vi "Call DQMH Scripting Tools.vi"(8 "error in":errorcluster, 9 "DQMH Tools":T2, 10 "Current Selection In":T1, 11 "Project in":refnum<class "Project.lvclass">) -> (0 "error out":errorcluster)   [LabVIEW 2020, in "Panther Dashboard.lvlib"]
uses:
  Panther Dashboard.lvlib
  Class/Project/Project.lvclass
  C:/GitClones/PantherDashboard/src/LabVIEW/Panther Dashboard/Class/LabVIEWItem/LabVIEWItem.lvclass
  DQMH Tools Menu--enum.ctl
  Class/Library/Library.lvclass
  Class/VI/VI.lvclass
  Class/Project/Project.lvclass/Project.ctl
  Class/LabVIEWItem/LabVIEWItem.lvclass/LabVIEWItem.ctl
  Class/LabVIEWItem/Read Item Type.vi
  Class/LabVIEWItem/Read Item Name.vi
  Class/Project/Read Main App Inst Ref.vi
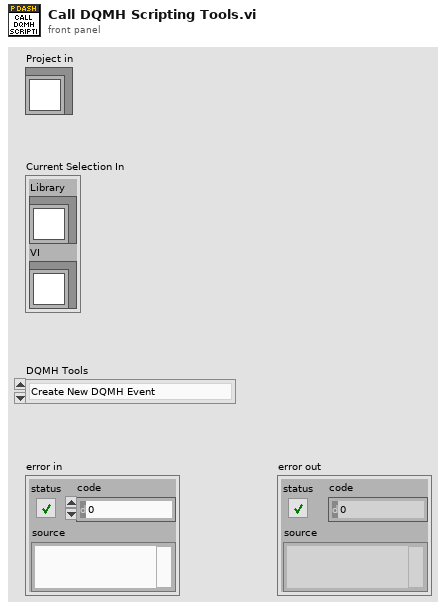
[diagram p1: front panel]
types:
  T1 = cluster{"Library":refnum<class "Library.lvclass">, "VI":refnum<class "VI.lvclass">}
  T2 = typedef "Panther Dashboard.lvlib/DQMH Tools Menu--enum.ctl" = enum16{"Create New DQMH Event", "Remove DQMH Event", "Convert DQMH Event", "Rename DQMH Event", "Add New DQMH Module", "Create RT Tester", "Rename DQMH Module", "Validate DQMH Module", "Create DQMH Module Template", "New DQMH  Unit Test", "Add Helper Loop to DQMH Module", "Duplicate Event", "Duplicate Module"}
  T3 = enum32{"Invalid", "Standard", "Closed", "Hidden", "Minimized", "Maximized"}
  T4 = typedef "Panther Dashboard.lvlib/LabVIEWItem.lvclass/Item Type--enum.ctl" = enum16{"Requests", "Broadcasts", "Request and Wait for Reply", "Round Trip", "» Public API VIs", "» Constant VIs", "» Error VIs", "Module", "Project", "No Drag Selection"}
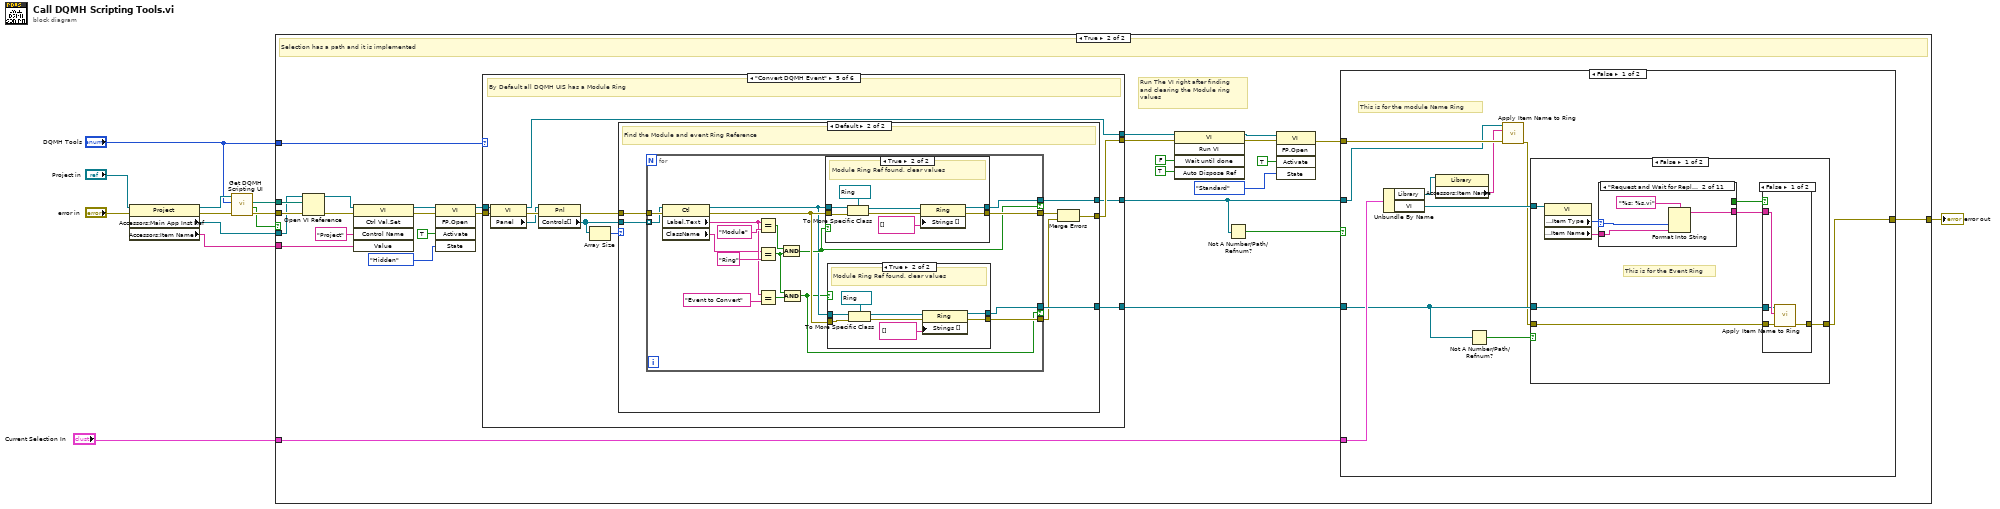
[diagram p0: block diagram]
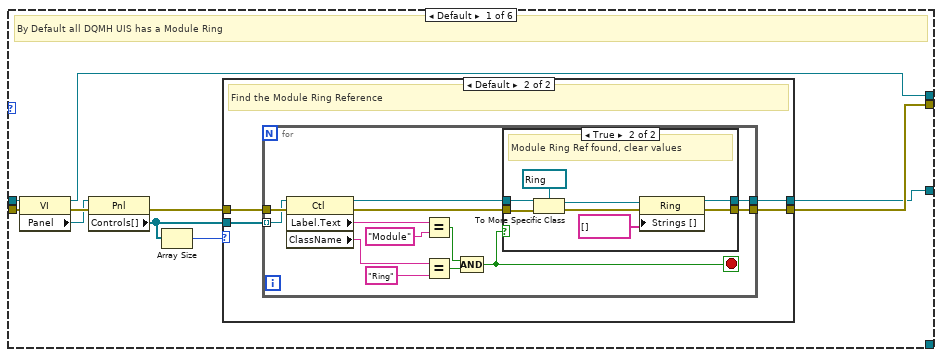
[diagram p3: hidden frame]
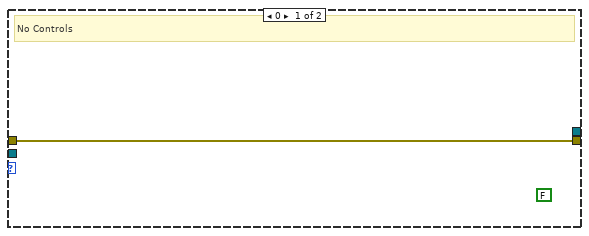
[diagram p4: hidden frame]
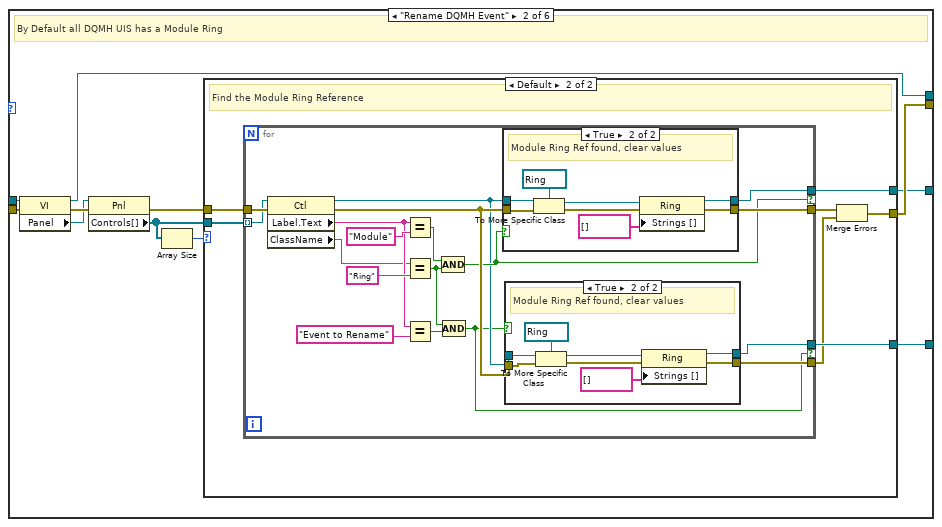
[diagram p6: hidden frame]
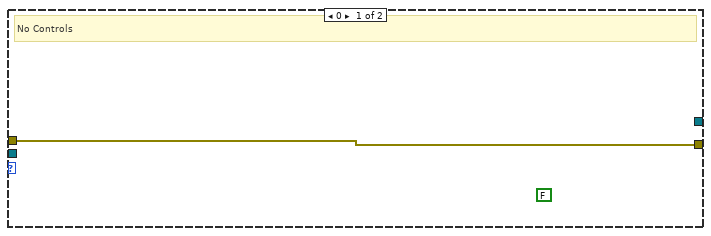
[diagram p7: hidden frame]
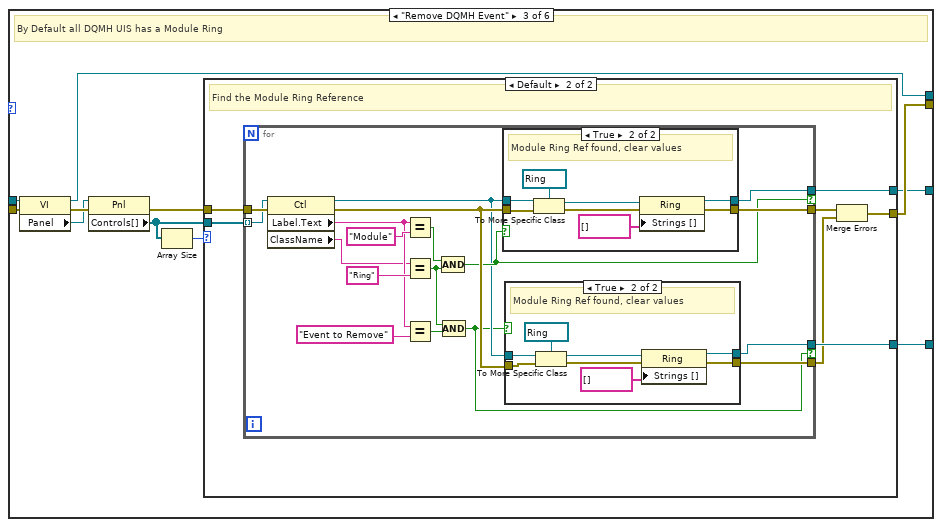
[diagram p10: hidden frame]
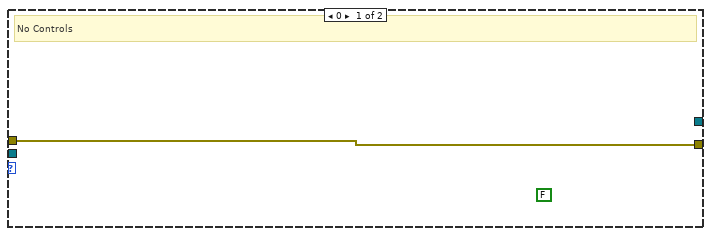
[diagram p11: hidden frame]
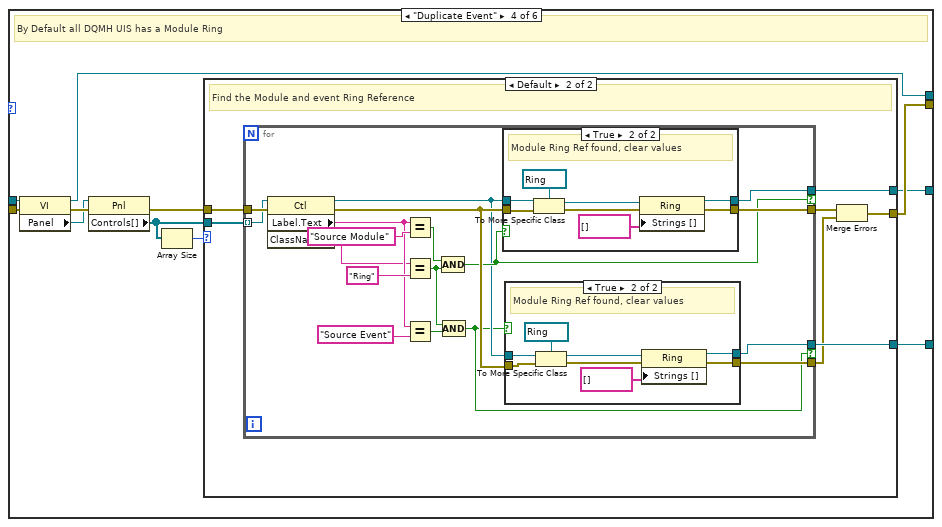
[diagram p14: hidden frame]
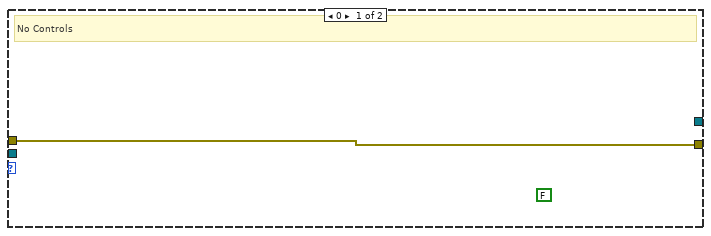
[diagram p15: hidden frame]
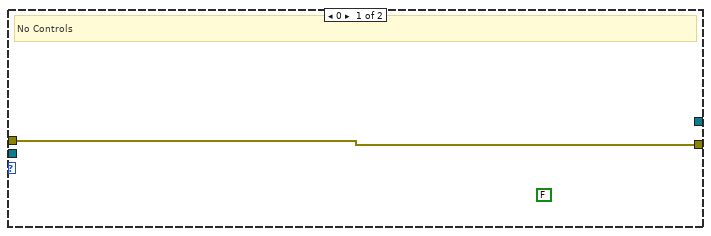
[diagram p18: hidden frame]
diagram:
  n1 = property class="Project"(reference="Project in", error in="error in") -> (reference out=w5:refnum<class "Project.lvclass">, error out=w9:errorcluster, "Accessors:Main App Inst Ref"=w4:refnum<vi>, "Accessors:Item Name"=w3:string)
  n2 = call "Get DQMH Scripting UI.vi"("error in"=w9, "DQMH Tools"="DQMH Tools", "Project in"=w5) -> ("error out"=w12:errorcluster, "Implemented?"=w7:bool, "DQMH UI Path"=w8:path)  [unwired: 6 in]
  n3 = case shown="True" w7 {
    tunnel: w8 -> [_ w32]
    tunnel: w3 -> [_ w27]
    tunnel: [w13 w34] -> w10
    tunnel: w12 -> [w13 w35]
    tunnel: w4 -> [_ w19]
    tunnel: "DQMH Tools" -> [_ w16]
    tunnel: "Current Selection In" -> [_ w15]
    frame False {
      # "Not Implemented"
    }
    frame True {
      # "Run The VI right after finding\nand clearing the Module ring\nvalues"
      # "Selection has a path and it is implemented"
      n4 = Open VI Reference(application reference (local)=w19, vi path=w32, error in (no error)=w35) -> (vi reference=w20:refnum<vi>, error out=w41:errorcluster)  [unwired: 3 in]
      n5 = invoke class="VI" method="Ctrl Val.Set"(reference=w20, error in=w41, "Control Name"="Project", "Value"=w27) -> (reference out=w25:refnum<vi>, error out=w39:errorcluster)  [unwired: 1 in, 3 out]
      n6 = invoke class="VI" method="FP.Open"(reference=w25, error in=w39, "Activate"=TRUE ("Activate?"), "State"=T3."Hidden") -> (reference out=w26:refnum<vi>, error out=w40:errorcluster)  [unwired: 1 in, 3 out]
      n7 = case shown="\"Convert DQMH Event\"" w16 {
        tunnel: w40 -> [w49 w87 w141 w195 w249 w296]
        tunnel: [w48 w86 w140 w194 w248 w296] -> w38
        tunnel: [w44 w82 w136 w190 w244 _] -> w18
        tunnel: w26 -> [w43 w81 w135 w189 w243 w295]
        tunnel: [w42 w80 w134 w188 w242 w295] -> w24
        tunnel: [_ w79 w133 w187 w241 _] -> w14
        frame Default {
          # "By Default all DQMH UIS has a Module Ring"
          n8 = property class="VI"(reference=w43, error in=w49) -> (reference out=w42:refnum<vi>, error out=w51:errorcluster, "Panel"=w47:refnum<vi>)
          n9 = property class="Pnl"(reference=w47, error in=w51) -> (error out=w50:errorcluster, "Controls[]"=w46:refnum<vi>[])  [unwired: 1 out]
          n10 = Array Size(array=w46) -> (size(s)=w45:i32)
          n11 = case shown="Default" w45 {
            tunnel: [_ w54] -> w44
            tunnel: w50 -> [w52 w56]
            tunnel: [w52 w55] -> w48
            tunnel: w46 -> [_ w53]
            frame 0 {
              (unwired) FALSE
              # "No Controls"
            }
            frame Default {
              # "Find the Module Ring Reference"
              n12 = for {
                tunnel: w53 -> [w66] mode=indexing
                tunnel: [w58] -> w54
                tunnel: w56 -> [w69]
                tunnel: [w67] -> w55
                stop <- w57 stop-if-true
                n13 = property class="Ctl"(reference=w66, error in=w69) -> (reference out=w59:refnum<vi>, error out=w68:errorcluster, "Label.Text"=w65:string, "ClassName"=w63:string)
                n14 = Equal?(x=w65, y="Module" ("Control Name")) -> (x = y?=w61:bool)
                n15 = Equal?(x=w63, y="Ring" ("Class Name")) -> (x = y?=w60:bool)
                n16 = Compound Arithmetic op=AND(w61, w60) -> (w57:bool)
                n17 = case shown="True" w57 {
                  tunnel: w68 -> [w70 w77]
                  tunnel: [w70 w78] -> w67
                  tunnel: w59 -> [_ w73]
                  tunnel: [_ w75] -> w58
                  frame False {
                  }
                  frame True {
                    # "Module Ring Ref found, clear values"
                    n18 = To More Specific Class(target class=refnum<vi> refnum ("Module"), reference=w73, error in=w77) -> (specific class reference=w72:refnum<vi>, error out=w76:errorcluster)
                    n19 = property class="Ring"(reference=w72, error in=w76, "Strings []"=string[] []) -> (reference out=w75:refnum<vi>, error out=w78:errorcluster)
                  }
                }
              }
            }
          }
        }
        frame "Rename DQMH Event" {
          # "By Default all DQMH UIS has a Module Ring"
          n20 = property class="VI"(reference=w81, error in=w87) -> (reference out=w80:refnum<vi>, error out=w89:errorcluster, "Panel"=w85:refnum<vi>)
          n21 = property class="Pnl"(reference=w85, error in=w89) -> (error out=w88:errorcluster, "Controls[]"=w84:refnum<vi>[])  [unwired: 1 out]
          n22 = Array Size(array=w84) -> (size(s)=w83:i32)
          n23 = case shown="Default" w83 {
            tunnel: [_ w95] -> w82
            tunnel: w88 -> [w90 w97]
            tunnel: [w90 w92] -> w86
            tunnel: w84 -> [_ w94]
            tunnel: [_ w93] -> w79
            frame 0 {
              (unwired) FALSE
              # "No Controls"
            }
            frame Default {
              # "Find the Module Ring Reference"
              n24 = for {
                tunnel: w94 -> [w111] mode=indexing
                tunnel: [w107] -> w95 if=w103
                tunnel: w97 -> [w115]
                tunnel: [w114] -> w96
                tunnel: [w101] -> w93 if=w100
                tunnel: [w112] -> w91
                n25 = property class="Ctl"(reference=w111, error in=w115) -> (reference out=w102:refnum<vi>, error out=w113:errorcluster, "Label.Text"=w99:string, "ClassName"=w98:string)
                n26 = Equal?(x=w99, y="Module" ("Control Name")) -> (x = y?=w108:bool)
                n27 = Equal?(x=w98, y="Ring" ("Class Name")) -> (x = y?=w106:bool)
                n28 = Equal?(x=w99, y="Event to Rename" ("Control Name")) -> (x = y?=w104:bool)
                n29 = Compound Arithmetic op=AND(w108, w106) -> (w103:bool)
                n30 = Compound Arithmetic op=AND(w106, w104) -> (w100:bool)
                n31 = case shown="True" w103 {
                  tunnel: w113 -> [w124 w131]
                  tunnel: [w124 w132] -> w114
                  tunnel: w102 -> [_ w127]
                  tunnel: [_ w129] -> w107
                  frame False {
                  }
                  frame True {
                    # "Module Ring Ref found, clear values"
                    n32 = To More Specific Class(target class=refnum<vi> refnum ("Module"), reference=w127, error in=w131) -> (specific class reference=w126:refnum<vi>, error out=w130:errorcluster)
                    n33 = property class="Ring"(reference=w126, error in=w130, "Strings []"=string[] []) -> (reference out=w129:refnum<vi>, error out=w132:errorcluster)
                  }
                }
                n34 = case shown="True" w100 {
                  tunnel: [_ w123] -> w112
                  tunnel: [_ w120] -> w101
                  tunnel: w102 -> [_ w116]
                  tunnel: w113 -> [_ w121]
                  frame False {
                  }
                  frame True {
                    # "Module Ring Ref found, clear values"
                    n35 = To More Specific Class(target class=refnum<vi> refnum ("Module"), reference=w116, error in=w121) -> (specific class reference=w118:refnum<vi>, error out=w122:errorcluster)
                    n36 = property class="Ring"(reference=w118, error in=w122, "Strings []"=string[] []) -> (reference out=w120:refnum<vi>, error out=w123:errorcluster)
                  }
                }
              }
              n37 = Merge Errors(w96, w91) -> (w92:errorcluster)
            }
          }
        }
        frame "Remove DQMH Event" {
          # "By Default all DQMH UIS has a Module Ring"
          n38 = property class="VI"(reference=w135, error in=w141) -> (reference out=w134:refnum<vi>, error out=w143:errorcluster, "Panel"=w139:refnum<vi>)
          n39 = property class="Pnl"(reference=w139, error in=w143) -> (error out=w142:errorcluster, "Controls[]"=w138:refnum<vi>[])  [unwired: 1 out]
          n40 = Array Size(array=w138) -> (size(s)=w137:i32)
          n41 = case shown="Default" w137 {
            tunnel: [_ w149] -> w136
            tunnel: w142 -> [w144 w151]
            tunnel: [w144 w146] -> w140
            tunnel: w138 -> [_ w148]
            tunnel: [_ w147] -> w133
            frame 0 {
              (unwired) FALSE
              # "No Controls"
            }
            frame Default {
              # "Find the Module Ring Reference"
              n42 = for {
                tunnel: w148 -> [w165] mode=indexing
                tunnel: [w161] -> w149 if=w157
                tunnel: w151 -> [w169]
                tunnel: [w168] -> w150
                tunnel: [w155] -> w147 if=w154
                tunnel: [w166] -> w145
                n43 = property class="Ctl"(reference=w165, error in=w169) -> (reference out=w156:refnum<vi>, error out=w167:errorcluster, "Label.Text"=w153:string, "ClassName"=w152:string)
                n44 = Equal?(x=w153, y="Module" ("Control Name")) -> (x = y?=w162:bool)
                n45 = Equal?(x=w152, y="Ring" ("Class Name")) -> (x = y?=w160:bool)
                n46 = Equal?(x=w153, y="Event to Remove" ("Control Name")) -> (x = y?=w158:bool)
                n47 = Compound Arithmetic op=AND(w162, w160) -> (w157:bool)
                n48 = Compound Arithmetic op=AND(w160, w158) -> (w154:bool)
                n49 = case shown="True" w157 {
                  tunnel: w167 -> [w178 w185]
                  tunnel: [w178 w186] -> w168
                  tunnel: w156 -> [_ w181]
                  tunnel: [_ w183] -> w161
                  frame False {
                  }
                  frame True {
                    # "Module Ring Ref found, clear values"
                    n50 = To More Specific Class(target class=refnum<vi> refnum ("Module"), reference=w181, error in=w185) -> (specific class reference=w180:refnum<vi>, error out=w184:errorcluster)
                    n51 = property class="Ring"(reference=w180, error in=w184, "Strings []"=string[] []) -> (reference out=w183:refnum<vi>, error out=w186:errorcluster)
                  }
                }
                n52 = case shown="True" w154 {
                  tunnel: [_ w177] -> w166
                  tunnel: [_ w174] -> w155
                  tunnel: w156 -> [_ w170]
                  tunnel: w167 -> [_ w175]
                  frame False {
                  }
                  frame True {
                    # "Module Ring Ref found, clear values"
                    n53 = To More Specific Class(target class=refnum<vi> refnum ("Module"), reference=w170, error in=w175) -> (specific class reference=w172:refnum<vi>, error out=w176:errorcluster)
                    n54 = property class="Ring"(reference=w172, error in=w176, "Strings []"=string[] []) -> (reference out=w174:refnum<vi>, error out=w177:errorcluster)
                  }
                }
              }
              n55 = Merge Errors(w150, w145) -> (w146:errorcluster)
            }
          }
        }
        frame "Duplicate Event" {
          # "By Default all DQMH UIS has a Module Ring"
          n56 = property class="VI"(reference=w189, error in=w195) -> (reference out=w188:refnum<vi>, error out=w197:errorcluster, "Panel"=w193:refnum<vi>)
          n57 = property class="Pnl"(reference=w193, error in=w197) -> (error out=w196:errorcluster, "Controls[]"=w192:refnum<vi>[])  [unwired: 1 out]
          n58 = Array Size(array=w192) -> (size(s)=w191:i32)
          n59 = case shown="Default" w191 {
            tunnel: [_ w203] -> w190
            tunnel: w196 -> [w198 w205]
            tunnel: [w198 w200] -> w194
            tunnel: w192 -> [_ w202]
            tunnel: [_ w201] -> w187
            frame 0 {
              (unwired) FALSE
              # "No Controls"
            }
            frame Default {
              # "Find the Module and event Ring Reference"
              n60 = for {
                tunnel: w202 -> [w219] mode=indexing
                tunnel: [w215] -> w203 if=w211
                tunnel: w205 -> [w223]
                tunnel: [w222] -> w204
                tunnel: [w209] -> w201 if=w208
                tunnel: [w220] -> w199
                n61 = property class="Ctl"(reference=w219, error in=w223) -> (reference out=w210:refnum<vi>, error out=w221:errorcluster, "Label.Text"=w207:string, "ClassName"=w206:string)
                n62 = Equal?(x=w207, y="Source Module" ("Control Name")) -> (x = y?=w216:bool)
                n63 = Equal?(x=w206, y="Ring" ("Class Name")) -> (x = y?=w214:bool)
                n64 = Equal?(x=w207, y="Source Event" ("Control Name")) -> (x = y?=w212:bool)
                n65 = Compound Arithmetic op=AND(w216, w214) -> (w211:bool)
                n66 = Compound Arithmetic op=AND(w214, w212) -> (w208:bool)
                n67 = case shown="True" w211 {
                  tunnel: w221 -> [w232 w239]
                  tunnel: [w232 w240] -> w222
                  tunnel: w210 -> [_ w235]
                  tunnel: [_ w237] -> w215
                  frame False {
                  }
                  frame True {
                    # "Module Ring Ref found, clear values"
                    n68 = To More Specific Class(target class=refnum<vi> refnum ("Module"), reference=w235, error in=w239) -> (specific class reference=w234:refnum<vi>, error out=w238:errorcluster)
                    n69 = property class="Ring"(reference=w234, error in=w238, "Strings []"=string[] []) -> (reference out=w237:refnum<vi>, error out=w240:errorcluster)
                  }
                }
                n70 = case shown="True" w208 {
                  tunnel: [_ w231] -> w220
                  tunnel: [_ w228] -> w209
                  tunnel: w210 -> [_ w224]
                  tunnel: w221 -> [_ w229]
                  frame False {
                  }
                  frame True {
                    # "Module Ring Ref found, clear values"
                    n71 = To More Specific Class(target class=refnum<vi> refnum ("Module"), reference=w224, error in=w229) -> (specific class reference=w226:refnum<vi>, error out=w230:errorcluster)
                    n72 = property class="Ring"(reference=w226, error in=w230, "Strings []"=string[] []) -> (reference out=w228:refnum<vi>, error out=w231:errorcluster)
                  }
                }
              }
              n73 = Merge Errors(w204, w199) -> (w200:errorcluster)
            }
          }
        }
        frame "Convert DQMH Event" {
          # "By Default all DQMH UIS has a Module Ring"
          n74 = property class="VI"(reference=w243, error in=w249) -> (reference out=w242:refnum<vi>, error out=w251:errorcluster, "Panel"=w247:refnum<vi>)
          n75 = property class="Pnl"(reference=w247, error in=w251) -> (error out=w250:errorcluster, "Controls[]"=w246:refnum<vi>[])  [unwired: 1 out]
          n76 = Array Size(array=w246) -> (size(s)=w245:i32)
          n77 = case shown="Default" w245 {
            tunnel: [_ w257] -> w244
            tunnel: w250 -> [w252 w259]
            tunnel: [w252 w254] -> w248
            tunnel: w246 -> [_ w256]
            tunnel: [_ w255] -> w241
            frame 0 {
              (unwired) FALSE
              # "No Controls"
            }
            frame Default {
              # "Find the Module and event Ring Reference"
              n78 = for {
                tunnel: w256 -> [w273] mode=indexing
                tunnel: [w269] -> w257 if=w265
                tunnel: w259 -> [w277]
                tunnel: [w276] -> w258
                tunnel: [w263] -> w255 if=w262
                tunnel: [w274] -> w253
                n79 = property class="Ctl"(reference=w273, error in=w277) -> (reference out=w264:refnum<vi>, error out=w275:errorcluster, "Label.Text"=w261:string, "ClassName"=w260:string)
                n80 = Equal?(x=w261, y="Module" ("Control Name")) -> (x = y?=w270:bool)
                n81 = Equal?(x=w260, y="Ring" ("Class Name")) -> (x = y?=w268:bool)
                n82 = Equal?(x=w261, y="Event to Convert" ("Control Name")) -> (x = y?=w266:bool)
                n83 = Compound Arithmetic op=AND(w270, w268) -> (w265:bool)
                n84 = Compound Arithmetic op=AND(w268, w266) -> (w262:bool)
                n85 = case shown="True" w265 {
                  tunnel: w275 -> [w286 w293]
                  tunnel: [w286 w294] -> w276
                  tunnel: w264 -> [_ w289]
                  tunnel: [_ w291] -> w269
                  frame False {
                  }
                  frame True {
                    # "Module Ring Ref found, clear values"
                    n86 = To More Specific Class(target class=refnum<vi> refnum ("Module"), reference=w289, error in=w293) -> (specific class reference=w288:refnum<vi>, error out=w292:errorcluster)
                    n87 = property class="Ring"(reference=w288, error in=w292, "Strings []"=string[] []) -> (reference out=w291:refnum<vi>, error out=w294:errorcluster)
                  }
                }
                n88 = case shown="True" w262 {
                  tunnel: [_ w285] -> w274
                  tunnel: [_ w282] -> w263
                  tunnel: w264 -> [_ w278]
                  tunnel: w275 -> [_ w283]
                  frame False {
                  }
                  frame True {
                    # "Module Ring Ref found, clear values"
                    n89 = To More Specific Class(target class=refnum<vi> refnum ("Module"), reference=w278, error in=w283) -> (specific class reference=w280:refnum<vi>, error out=w284:errorcluster)
                    n90 = property class="Ring"(reference=w280, error in=w284, "Strings []"=string[] []) -> (reference out=w282:refnum<vi>, error out=w285:errorcluster)
                  }
                }
              }
              n91 = Merge Errors(w258, w253) -> (w254:errorcluster)
            }
          }
        }
        frame "Add New DQMH Module" {
          # "No Module Ring In FP, do not search"
        }
      }
      n92 = invoke class="VI" method="Run VI"(reference=w24, error in=w38, "Wait until done"=FALSE ("Wait Until Done"), "Auto Dispose Ref"=TRUE ("Auto Dispose Reference")) -> (reference out=w22:refnum<vi>, error out=w37:errorcluster)  [unwired: 1 in, 3 out]
      n93 = Not A Number/Path/Refnum?(number/path/refnum=w18) -> (NaN/Path/Refnum?=w17:bool)
      n94 = invoke class="VI" method="FP.Open"(reference=w22, error in=w37, "Activate"=TRUE ("Activate?"), "State"=T3."Standard") -> (error out=w36:errorcluster)  [unwired: 1 in, 4 out]
      n95 = case shown="False" w17 {
        tunnel: w18 -> [w304 _]
        tunnel: w36 -> [w306 w333]
        tunnel: [w305 w333] -> w34
        tunnel: w15 -> [w301 _]
        tunnel: w14 -> [w298 _]
        frame False {
          # "This is for the module Name Ring"
          n96 = Unbundle By Name(w301) -> ("Library"=w302:refnum<class "Library.lvclass">, "VI"=w303:refnum<class "VI.lvclass">)
          n97 = property class="Library"(reference=w302) -> ("Accessors:Item Name"=w300:string)  [unwired: 1 in, 2 out]
          n98 = Not A Number/Path/Refnum?(number/path/refnum=w298) -> (NaN/Path/Refnum?=w299:bool)
          n99 = call "Apply Item Name to Ring.vi"("error in"=w306, "Item Name"=w300, "Ring in"=w304) -> ("error out"=w297:errorcluster)  [unwired: 8 in]
          n100 = case shown="False" w299 {
            tunnel: w303 -> [w312 _]
            tunnel: w298 -> [w309 _]
            tunnel: w297 -> [w314 _]
            tunnel: [w313 _] -> w305
            frame False {
              # "This is for the Event Ring"
              n101 = property class="VI"(reference=w312) -> ("Accessors:Item Type"=w311:T4, "Accessors:Item Name"=w310:string)  [unwired: 1 in, 2 out]
              n102 = case shown="\"Request and Wait for Reply\"" w311 {
                selector: w311 -> [_ w324 _ _ _ _ _ _ _ _ _]
                tunnel: [_ w322 w328 w332 _ _ _ _ _ _ _] -> w308
                tunnel: w310 -> [_ w321 w325 w329 _ _ _ _ _ _ _]
                tunnel: [TRUE _ _ _ _ _ _ _ _ _ _] -> w307
                frame Default {
                }
                frame "Request and Wait for Reply" {
                  n103 = Format Into String(format string="%s: %s.vi", w324, w321) -> (resulting string=w322:string)  [unwired: 2 in, 1 out]
                }
                frame "Broadcasts" {
                  n104 = Format Into String(format string="%s: %s.vi", "Broadcast" ("format string"), w325) -> (resulting string=w328:string)  [unwired: 2 in, 1 out]
                }
                frame "Requests" {
                  n105 = Format Into String(format string="%s: %s.vi", "Request" ("format string"), w329) -> (resulting string=w332:string)  [unwired: 2 in, 1 out]
                }
                frame "Round Trip" {
                }
                frame "» Public API VIs" {
                }
                frame "» Constant VIs" {
                }
                frame "» Error VIs" {
                }
                frame "Module" {
                }
                frame "Project" {
                }
                frame "No Drag Selection" {
                }
              }
              n106 = case shown="False" w307 {
                tunnel: w309 -> [w315 _]
                tunnel: w308 -> [w316 _]
                tunnel: w314 -> [w317 w319]
                tunnel: [w318 w319] -> w313
                frame False {
                  n107 = call "Apply Item Name to Ring.vi"("error in"=w317, "Item Name"=w316, "Ring in"=w315) -> ("error out"=w318:errorcluster)  [unwired: 8 in]
                }
                frame True {
                }
              }
            }
            frame True {
            }
          }
        }
        frame True {
          # "Null Reference, do nothing"
        }
      }
    }
  }
  "error out" <- w10
